vi "Initialize - Device Properties.vi"(8 "error in (no error)":errorcluster, 11 "Device Item Ref in":T1 format="%.0x") -> (0 "error out":errorcluster, 3 "Item Ref out":T1 format="%.0x")   [LabVIEW 2019, in "UDP-Custom-Device System Explorer.lvlib"]
doc: "Initialize the UDP Data Link custom device properties."
uses:
  UDP-Custom-Device System Explorer.lvlib
  <vilib>/NI VeriStand/Custom Device API/Custom Device Item Ref.ctl
  Property Accessors/Main Accessors.lvlib
  <vilib>/NI VeriStand/Custom Device API/Custom Device API.lvlib
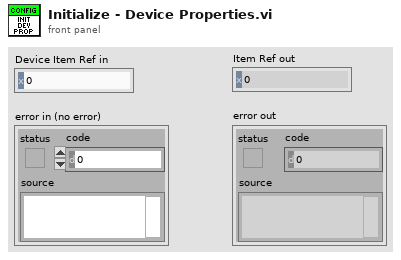
[diagram p1: front panel]
types:
  T1 = typedef "Custom Device API.lvlib/Custom Device Item Ref.ctl" = u64
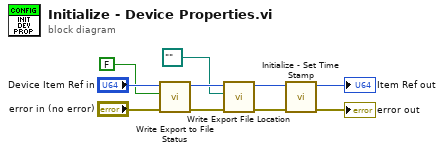
[diagram p0: block diagram]
diagram:
  n1 = call "Write Export to File Status.vi"("error in (no error)"="error in (no error)", "Export to File Status"=FALSE ("Value"), "Node Ptr"="Device Item Ref in") -> ("error out"=w5:errorcluster, "Node Ptr out"=w6:T1)  [unwired: 7 in]
  n2 = call "Write Export File Location.vi"("error in (no error)"=w5, "Export File Location"=path "" ("Value"), "Node Ptr"=w6) -> ("error out"=w3:errorcluster, "Node Ptr out"=w4:T1)  [unwired: 7 in]
  n3 = call "Initialize - Set Time Stamp.vi"("error in (no error)"=w3, "Device Item Ref in"=w4) -> ("error out"=→"error out":errorcluster, "Device Item Ref out"=→"Item Ref out":T1)  [unwired: 7 in, 1 out]
